vi "Main.vi"(8 "error in":errorcluster, 11 "Manager Panel in":refnum<class "Manager Panel.lvclass">) -> (0 "error out":errorcluster, 3 "Manager Panel out":refnum<class "Manager Panel.lvclass">)   [LabVIEW 2020, in "Manager Panel.lvclass"]
doc: "The <b>Queued Message Handler</b> of the Worker that owns this VI."
uses:
  Manager Panel.lvclass
  C:/Program Files (x86)/National Instruments/LabVIEW 2020/vi.lib/addons/_Workers/Library/Classes/Worker/Worker.lvclass
  Manager Panel.lvclass/Manager Panel.ctl
  Base Classes/BaseView/rqp_InsertPanel.ctl
  Initialization Data.ctl
  Response Cases.ctl
  ChartView/ChartView.lvclass
  C:/Users/kevin/Desktop/Workers5.0_1/Workers/Base Classes/BaseView/BaseView.lvclass
  ConfigView/ConfigView.lvclass
  LoginView/LoginView.lvclass
  <vilib>/addons/_Workers/Library/Classes/Message Queue/Message Queue.lvclass
  Base Classes/BaseView/BaseView.lvclass
panel:
  in  "ButtonMenu":enum32{"ChartView", "Config", "User"}(radio)
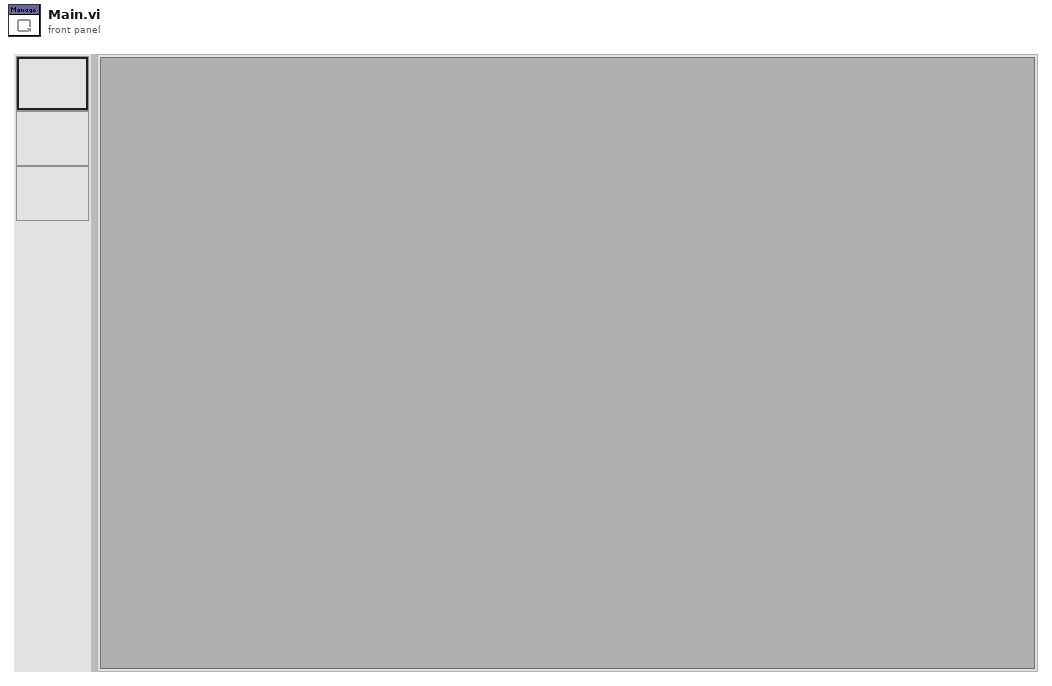
[diagram p1: front panel]
types:
  T1 = typedef "Manager Panel.lvclass/Initialization Data.ctl" = cluster{"Response Cases":T2}
  T2 = typedef "Manager Panel.lvclass/Response Cases.ctl" = cluster{"Placeholder - Can be deleted":string}
  T3 = typedef "BaseView.lvclass/rqp_InsertPanel.ctl" = cluster{"SubPanel":refnum<vi>}
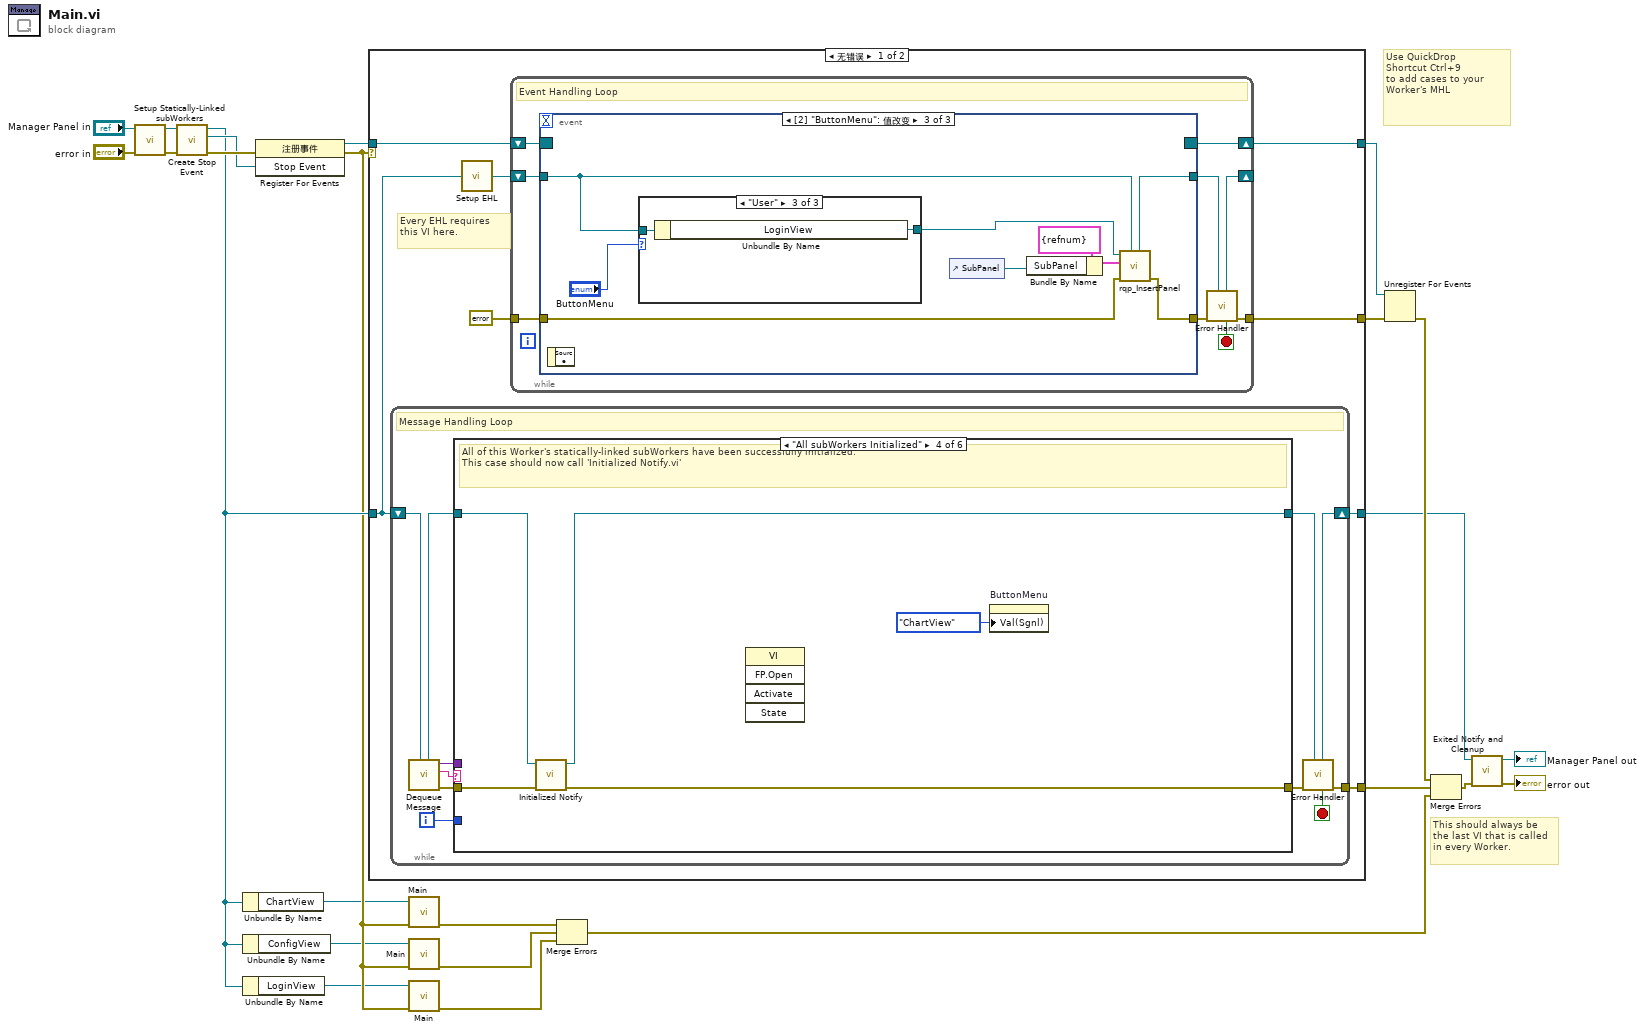
[diagram p0: block diagram]
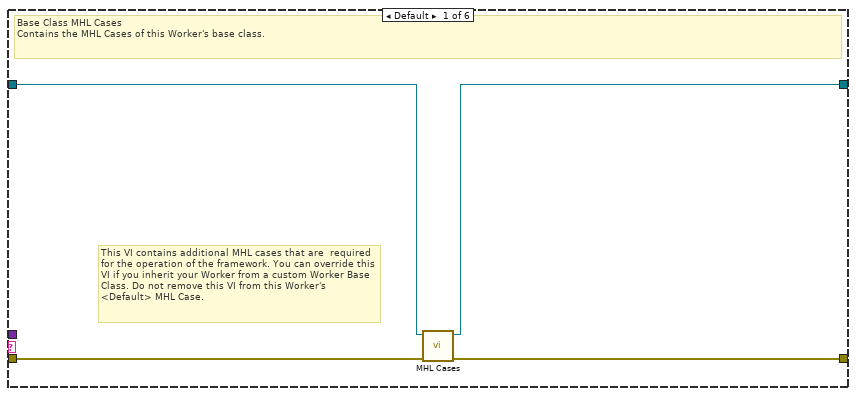
[diagram p2: hidden frame]
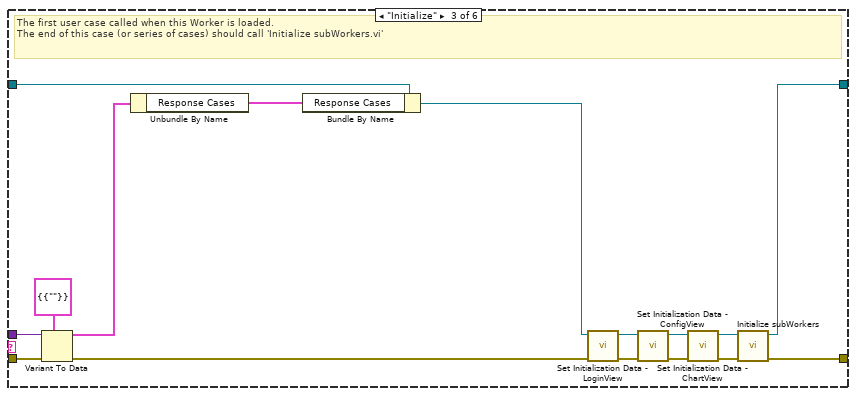
[diagram p4: hidden frame]
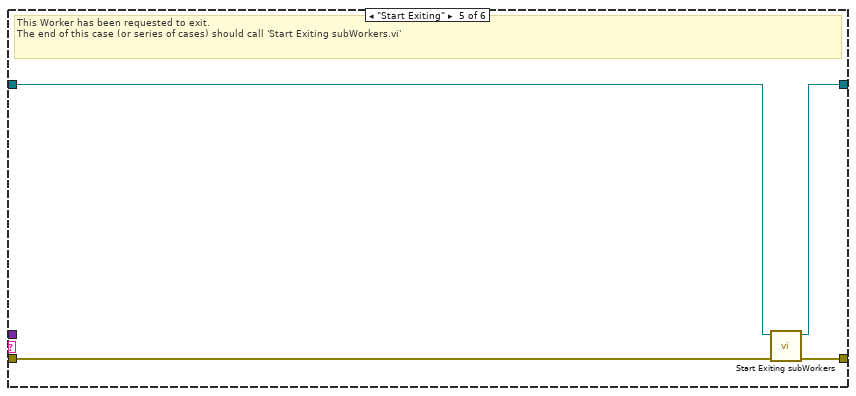
[diagram p5: hidden frame]
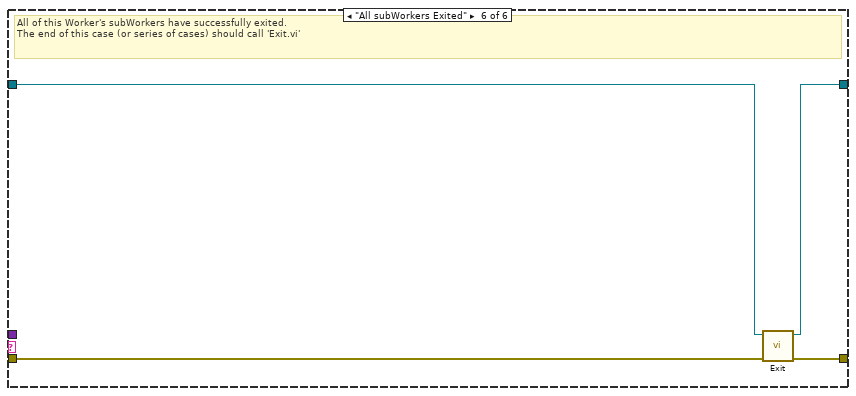
[diagram p6: hidden frame]
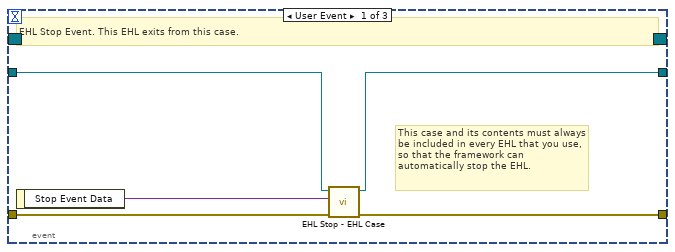
[diagram p7: hidden frame]
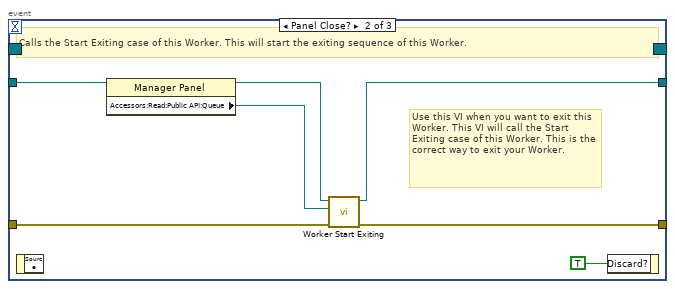
[diagram p8: hidden frame]
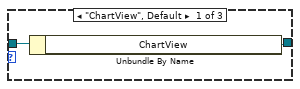
[diagram p9: hidden frame]
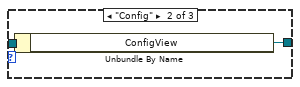
[diagram p10: hidden frame]
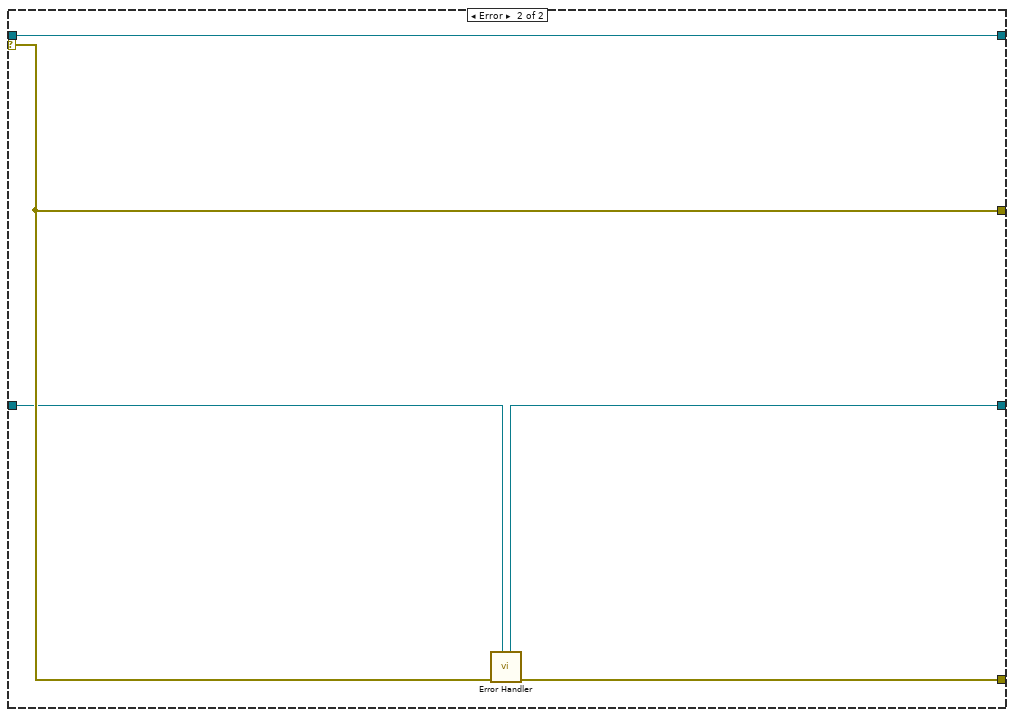
[diagram p11: hidden frame]
diagram:
  # "Use QuickDrop\nShortcut Ctrl+9\nto add cases to your\nWorker's MHL"
  # "This should always be the last VI that is called in every Worker."
  n1 = call "Setup Statically-Linked subWorkers.vi"("error in"="error in", "Manager Panel in"="Manager Panel in") -> ("error out"=w10:errorcluster, "Manager Panel out"=w8:refnum<class "Manager Panel.lvclass">)  [unwired: 8 in]
  n2 = call-dynamic "Create Stop Event.vi"("error in"=w10, "Worker"=w8) -> ("error out"=w19:errorcluster, "Stop Event"=w16:refnum<user-event>, "Worker out"=w13:refnum<class "Manager Panel.lvclass">)  [unwired: 7 in]
  n3 = Unbundle By Name(w13) -> ("ChartView"=w5:refnum<class "ChartView.lvclass">)
  n4 = Unbundle By Name(w13) -> ("ConfigView"=w3:refnum<class "ConfigView.lvclass">)
  n5 = Unbundle By Name(w13) -> ("LoginView"=w1:refnum<class "LoginView.lvclass">)
  n6 = register-events(error in=w19, w16) -> (reference out=w18:refnum<event-registration>, error out=w11:errorcluster)  [unwired: 1 in]
  n7 = case shown="无错误" w11 {
    tunnel: w13 -> [w27 w116]
    tunnel: [w25 w117] -> w17
    tunnel: w18 -> [w32 w118]
    tunnel: [w29 w119] -> w23
    tunnel: [w31 w118] -> w22
    tunnel: [w26 w115] -> w20
    selector: w11 -> [_ w119]
    frame No Error {
      # "Every EHL requires\nthis VI here."
      n8 = while {
        shift-right: [w41] -> w26
        shift-left: w27 -> [w43]
        tunnel: [w42] -> w25
        i -> [w33]
        stop <- w34 stop-if-true
        # "Message Handling Loop"
        n9 = call-dynamic "Dequeue Message.vi"("Worker"=w43) -> ("error out"=w40:errorcluster, "Case out"=w35:string, "Data out"=w36:variant, "Worker out"=w38:refnum<class "Manager Panel.lvclass">)  [unwired: 6 in, 1 out]
        n10 = case "Worker MHL Case Structure (DO NOT CHANGE LABEL NAME)" shown="\"All subWorkers Initialized\"" w35 {
          tunnel: w40 -> [w47 w48 w63 w68 w71 w78]
          tunnel: [w46 w48 w65 w67 w74 w77] -> w39
          tunnel: w38 -> [w45 w49 w62 w70 w72 w76]
          tunnel: [w44 w49 w64 w69 w73 w75] -> w37
          tunnel: w36 -> [_ _ w60 _ _ _]
          tunnel: w33 -> [_ _ _ _ _ _]
          frame Default {
            # "This VI contains additional MHL cases that are  required for the operation of the framework. You can override this VI if you inherit your Worker from a custom Worker Base Class. Do not remove this VI from this Worker's <Default> MHL Case."
            # "Base Class MHL Cases\nContains the MHL Cases of this Worker's base class."
            n11 = call-dynamic "MHL Cases.vi"("error in"=w47, "Worker in"=w45) -> ("error out"=w46:errorcluster, "Worker out"=w44:refnum<class "Manager Panel.lvclass">)  [unwired: 8 in]
          }
          frame "------------ FRAMEWORK CASES -----------" {
            # "Start of Workers Framework Cases"
          }
          frame "Initialize" {
            # "The first user case called when this Worker is loaded.\nThe end of this case (or series of cases) should call 'Initialize subWorkers.vi'"
            n12 = Variant To Data(error in=w63, type=T1 {"Response Cases"={"Placeholder - Can be deleted"=""}} ("Initialization Data"), Variant=w60) -> (data=w59:T1, error out=w61:errorcluster)
            n13 = Unbundle By Name(w59) -> ("Response Cases"=w58:T2)
            n14 = Bundle By Name ("按名称捆绑")(cluster=w62, "Response Cases"=w58) -> (w51:refnum<class "Manager Panel.lvclass">)
            n15 = call "Set Initialization Data - LoginView.vi"("error in"=w61, "Manager Panel in"=w51) -> ("error out"=w52:errorcluster, "Manager Panel out"=w50:refnum<class "Manager Panel.lvclass">)  [unwired: 8 in]
            n16 = call "Set Initialization Data - ConfigView.vi"("error in"=w52, "Manager Panel in"=w50) -> ("error out"=w54:errorcluster, "Manager Panel out"=w53:refnum<class "Manager Panel.lvclass">)  [unwired: 8 in]
            n17 = call "Set Initialization Data - ChartView.vi"("error in"=w54, "Manager Panel in"=w53) -> ("error out"=w56:errorcluster, "Manager Panel out"=w55:refnum<class "Manager Panel.lvclass">)  [unwired: 8 in]
            n18 = call-dynamic "Initialize subWorkers.vi"("error in"=w56, "Worker"=w55) -> ("error out"=w65:errorcluster, "dup Worker out"=w64:refnum<class "Manager Panel.lvclass">)  [unwired: 8 in]
          }
          frame "All subWorkers Initialized" {
            # "All of this Worker's statically-linked subWorkers have been successfully initialized.\nThis case should now call 'Initialized Notify.vi'"
            n19 = call-dynamic "Initialized Notify.vi"("error in"=w68, "Worker"=w70) -> ("error out"=w67:errorcluster, "dup Worker out"=w69:refnum<class "Manager Panel.lvclass">)  [unwired: 8 in]
            n20 = invoke class="VI" method="FP.Open"() -> ()  [unwired: 5 in, 5 out]
            n21 = property on="ButtonMenu" class="RadioBtnsControl (严格)"("Val(Sgnl)"=enum32{"ChartView", "Config", "User"}."ChartView" ("值(信号)")) -> ()  [unwired: 2 in, 2 out]
          }
          frame "Start Exiting" {
            # "This Worker has been requested to exit. \nThe end of this case (or series of cases) should call 'Start Exiting subWorkers.vi'"
            n22 = call-dynamic "Start Exiting subWorkers.vi"("error_in"=w71, "Worker"=w72) -> ("error out"=w74:errorcluster, "dup Worker out"=w73:refnum<class "Manager Panel.lvclass">)  [unwired: 8 in]
          }
          frame "All subWorkers Exited" {
            # "All of this Worker's subWorkers have successfully exited. \nThe end of this case (or series of cases) should call 'Exit.vi'"
            n23 = call-dynamic "Exit.vi"("error_in"=w78, "Worker"=w76) -> ("error out"=w77:errorcluster, "dup Worker out"=w75:refnum<class "Manager Panel.lvclass">)  [unwired: 8 in]
          }
        }
        n24 = call-dynamic "Error Handler.vi"("Worker"=w37, "error_in"=w39) -> ("error out"=w42:errorcluster, "Stop Loop"=w34:bool, "Worker out"=w41:refnum<class "Manager Panel.lvclass">)  [unwired: 7 in]
      }
      n25 = call-dynamic "Setup EHL.vi"("Worker"=w27) -> ("Worker out"=w28:refnum<class "Manager Panel.lvclass">)  [unwired: 14 in]
      n26 = while "Event Handling Loop" {
        shift-right: [w87] -> w31
        shift-left: w32 -> [w86]
        tunnel: [w82] -> w29
        tunnel: errorcluster {"status"=FALSE, "code"=0, "source"=""} ("error constant") -> [w84]
        shift-right: [w80] -> _
        shift-left: w28 -> [w85]
        stop <- w79 stop-if-true
        # "Event Handling Loop"
        n27 = event shown="[2] \"ButtonMenu\": 值改变" {
          selector: w86 -> [_ _ _]
          dyn-events: [_ _ _] -> w87
          timeout: _ -> [_ _ _]
          tunnel: [w91 w98 w103] -> w83
          tunnel: w84 -> [w92 w97 w104]
          tunnel: w85 -> [w90 w96 w102]
          tunnel: [w89 w95 w108] -> w81
          event User Event {
            # "This case and its contents must always be included in every EHL that you use, so that the framework can automatically stop the EHL."
            # "EHL Stop Event. This EHL exits from this case."
            n28 = event-data() -> ("Stop Event Data"=w88:variant)  [unwired: 1 in]
            n29 = call-dynamic "EHL Stop - EHL Case.vi"("error in"=w92, "Stop Event Data"=w88, "Worker"=w90) -> ("error out"=w91:errorcluster, "Worker out"=w89:refnum<class "Manager Panel.lvclass">)  [unwired: 7 in]
          }
          event Panel Close? {
            # "Use this VI when you want to exit this Worker. This VI will call the Start Exiting case of this Worker. This is the correct way to exit your Worker."
            # "Calls the Start Exiting case of this Worker. This will start the exiting sequence of this Worker."
            n30 = event-data() -> ()  [unwired: 1 in, 1 out]
            n31 = property class="Manager Panel"(reference=w96) -> (reference out=w94:refnum<class "Manager Panel.lvclass">, "Accessors:Read:Public API:Queue"=w93:refnum<class "Message Queue.lvclass">)  [unwired: 1 in, 1 out]
            n32 = call-dynamic "Worker Start Exiting.vi"("error_in"=w97, "Message Queue"=w93, "Worker"=w94) -> ("error out"=w98:errorcluster, "dup Worker out"=w95:refnum<class "Manager Panel.lvclass">)  [unwired: 7 in]
            n33 = event-data ("事件过滤节点")("Discard?"=TRUE) -> ()  [unwired: 1 in, 1 out]
          }
          event "ButtonMenu": Value Change {
            n34 = event-data() -> ()  [unwired: 1 in, 1 out]
            n35 = case shown="\"User\"" "ButtonMenu" {
              tunnel: w102 -> [w110 w112 w114]
              tunnel: [w109 w111 w113] -> w100
              frame "ChartView", Default {
                n36 = Unbundle By Name(w110) -> ("ChartView"=w109:refnum<class "ChartView.lvclass">)
              }
              frame "Config" {
                n37 = Unbundle By Name(w112) -> ("ConfigView"=w111:refnum<class "ConfigView.lvclass">)
              }
              frame "User" {
                n38 = Unbundle By Name(w114) -> ("LoginView"=w113:refnum<class "LoginView.lvclass">)
              }
            }
            n39 = control-ref of="SubPanel"() -> (w105:refnum<vi>)
            n40 = Bundle By Name(cluster=T3 {"SubPanel"=refnum} ("Data in"), "SubPanel"=w105) -> (w106:T3)
            n41 = call "rqp_InsertPanel.vi"("Caller in"=w102, "error in"=w104, "Data in"=w106, "BaseView in"=w100) -> ("error out"=w103:errorcluster, "dup Caller out"=w108:refnum<class "Manager Panel.lvclass">)  [unwired: 5 in, 1 out]
          }
        }
        n42 = call-dynamic "Error Handler.vi"("Worker"=w81, "error_in"=w83) -> ("error out"=w82:errorcluster, "Stop Loop"=w79:bool, "Worker out"=w80:refnum<class "Manager Panel.lvclass">)  [unwired: 7 in]
      }
    }
    frame Error {
      n43 = call-dynamic "Error Handler.vi"("Worker"=w116, "error_in"=w119) -> ("error out"=w117:errorcluster, "Worker out"=w115:refnum<class "Manager Panel.lvclass">)  [unwired: 7 in, 1 out]
    }
  }
  n44 = call-dynamic "Main.vi"("error in"=w11, "ChartView in"=w5) -> ("error out"=w7:errorcluster)  [unwired: 8 in, 1 out]
  n45 = call-dynamic "Main.vi"("error in"=w11, "ConfigView in"=w3) -> ("error out"=w4:errorcluster)  [unwired: 8 in, 1 out]
  n46 = call-dynamic "Main.vi"("error in"=w11, "LoginView in"=w1) -> ("error out"=w2:errorcluster)  [unwired: 8 in, 1 out]
  n47 = Merge Errors(w7, w4, w2) -> (w6:errorcluster)
  n48 = Unregister For Events(event registration refnum=w22, error in=w23) -> (error out=w24:errorcluster)
  n49 = Merge Errors ("合并错误")(w24, w17, w6) -> (w21:errorcluster)
  n50 = call-dynamic "Exited Notify and Cleanup.vi"("error_in"=w21, "Worker"=w20) -> ("error out"=→"error out":errorcluster, "dup Worker out"=→"Manager Panel out":refnum<class "Manager Panel.lvclass">)  [unwired: 8 in]
